vi "PV config A D input output.vi"(8 "error in (no error)":errorcluster, 9 "PV config A D input output - Cluster":T1={"Parameter"=enum." Configuration DO2 (019)", "Parameter\nread only<->describe"=FALSE, "off<->on   "=TRUE, "Configuration DO1 / DO2 / R1 / R2 / R3"=0, "Configuration AO1"=0, "Config. Acces. A1/A2"=0, "Config. Acces. B1/B2"=0, "Configuration DI1 / DI2 / DI3"=0} {"Configuration DI1 / DI2 / DI3" items=["0 = deactivated", "1 = enable venting", "2 = heating", "3 = sealing gas", "4 = run-up time control", "5 = rotation speed setting mode", "6 =", "7 = Sensor 1 HV enable"]; "Config. Acces. B1/B2" items=[" fan (continous operation) (default)", " venting valve, normally closed", " heating", " backing pump", " fan (temperature controlled)", " sealing gas", " always 0 (off)", " always 1 (on)", " power failure venting unit"]; "Config. Acces. A1/A2" items=[" fan (continous operation)", " venting valve, normally closed", " heating", " backing pump", " fan (temperature controlled)", " sealing gas", " always off", " always on", " power failure venting unit"]; "Configuration DO1 / DO2 / R1 / R2 / R3" items=["0 = rot. speed switch point attained", "1 = no error", "2 = error", "3 = warning", "4 = error and/or warning", "5 = set speed attained", "6 = pump on", "7 = pump accelerates", "8 = pump decelerater", "9 = always 0 (off)", "10 = always 1 (on)", "11 = remote priority active", "12 = heating", "13 = backing pump", "14 = sealing gas", "15 = pumping station", "16 = pump rotates", "17 = pump does not rotate", "18 = TMS temperature engaged  ", "19 = Pressure below pressure switchpoint 1", "20 = Pressure below pressure switchpoint 2"]; "Configuration AO1" items=["0 = actual rotation speed", "1 = power", "2 = current", "3 = always 0 V", "4 = always 10 V", "5 = follows AI1", "6 = Pressure value 1", "7 = Pressure value 2"]}, 10 "Adress of unit":u16=1 max=999 step=1, 11 "VISA session":refnum<visa-resource-name>) -> (0 "error out":errorcluster, 2 "response (data)":string, 3 "dup VISA session":refnum<visa-resource-name>)   [LabVIEW 2021, in "Pfeiffer Vacuum.lvlib"]
doc: "There are 15 parameters available, only one of which can be enabled at a time. \n\n Configuration DO2 (019)\n Configuration DO1 (024) \n Configuration heating output (032)\n Configuration accessory A1 (035)\n Configuration accessory B1 (036)\n Configuration accessory A2 (037)\n Configuration accessory B2 (038)\n Configuration Relais 1 (045)\n Configuration Relais 2 (046)\n Configuration Relais 3 (047)\n Configuration AO1 (055)\n Configuration AI1 (057)\n Configuration DI1 (062)\n Configuration DI2 (063)\n Configuration DI3 (064)\n\nNote: Any settings for an parameter that is not selected will be ignored. If a value is out of range, it will be changed to either the upper or the lower limit of the range."
uses:
  <instrlib>/Pfeiffer Vacuum/Pfeiffer Vacuum.lvlib
  <instrlib>/Pfeiffer Vacuum/Public/Turbopumps/PV config A D input output - Cluster.ctl
panel:
  # "<--------------                  ------------->     \n                                                                                        false                             true \n Configuration heating output K4    :                           heat/TMS            ealing gas valve control  \n Configuration AI 1                          :                            disabled                       set speed"
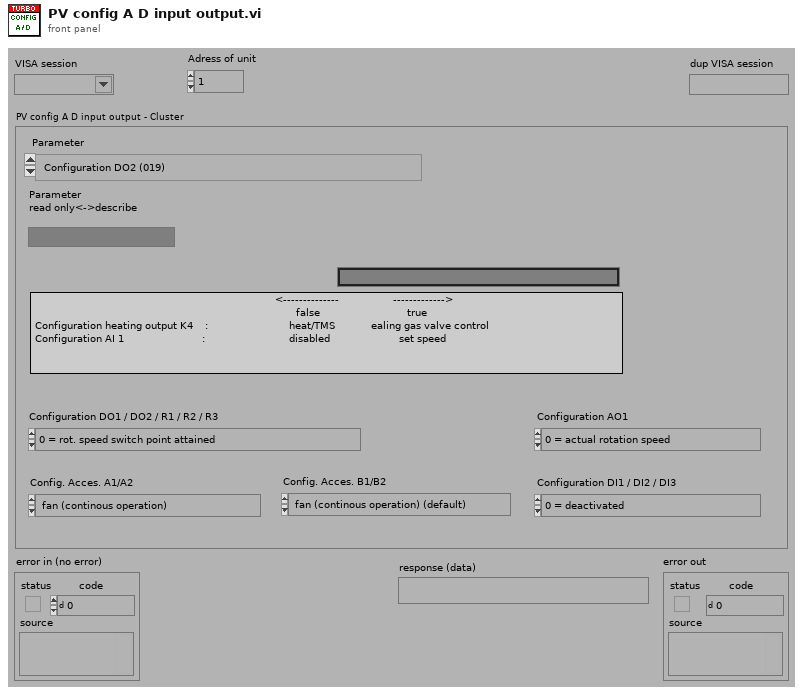
[diagram p1: front panel]
types:
  T1 = typedef "Pfeiffer Vacuum.lvlib/PV config A D input output - Cluster.ctl" = cluster{"Parameter":enum16{" Configuration DO2 (019)", " Configuration DO1 (024)", " Configuration heating output (032)", " Configuration accessory A1 (035)", " Configuration accessory B1 (036)", " Configuration accessory A2 (037)", " Configuration accessory B2 (038)", " Configuration Relais 1 (045)", " Configuration Relais 2 (046)", " Configuration Relais 3 (047)", " Configuration AO1 (055)", " Configuration AI1 (057)", " Configuration DI1 (062)", " Configuration DI2 (063)", " Configuration DI3 (064)"}, "Parameter\nread only<->describe":bool, "off<->on   ":bool, "Configuration DO1 / DO2 / R1 / R2 / R3":u16, "Configuration AO1":u16, "Config. Acces. A1/A2":u16, "Config. Acces. B1/B2":u16, "Configuration DI1 / DI2 / DI3":u16}
  T2 = enum16{" Configuration DO2 (019)", " Configuration DO1 (024)", " Configuration heating output (032)", " Configuration accessory A1 (035)", " Configuration accessory B1 (036)", " Configuration accessory A2 (037)", " Configuration accessory B2 (038)", " Configuration Relais 1 (045)", " Configuration Relais 2 (046)", " Configuration Relais 3 (047)", " Configuration AO1 (055)", " Configuration AI1 (057)", " Configuration DI1 (062)", " Configuration DI2 (063)", " Configuration DI3 (064)"}
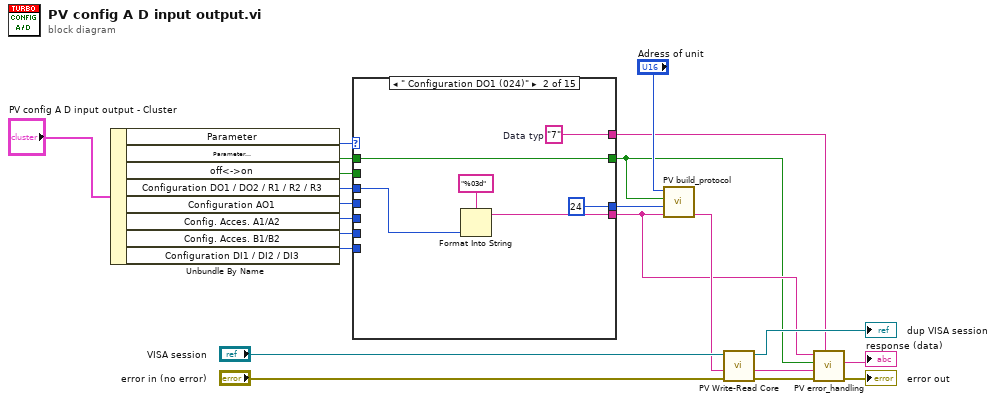
[diagram p0: block diagram]
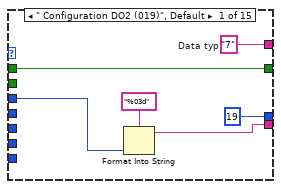
[diagram p2: hidden frame]
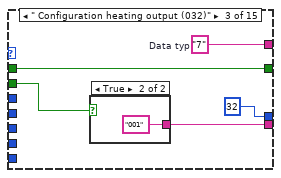
[diagram p3: hidden frame]
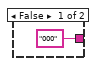
[diagram p4: hidden frame]
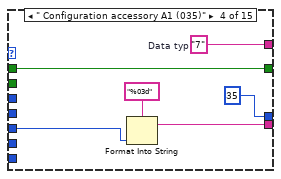
[diagram p5: hidden frame]
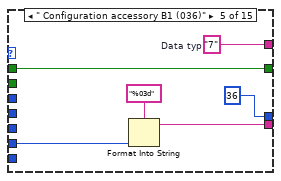
[diagram p6: hidden frame]
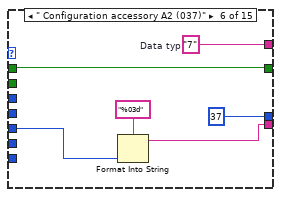
[diagram p7: hidden frame]
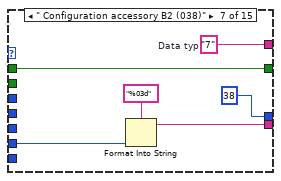
[diagram p8: hidden frame]
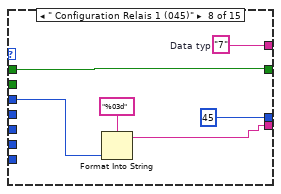
[diagram p9: hidden frame]
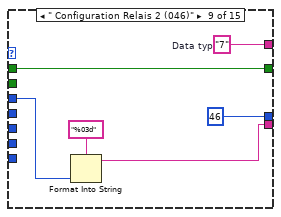
[diagram p10: hidden frame]
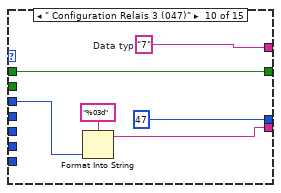
[diagram p11: hidden frame]
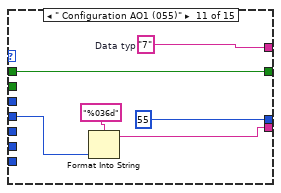
[diagram p12: hidden frame]
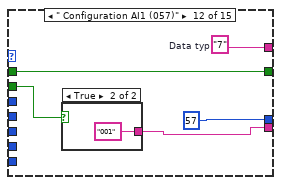
[diagram p13: hidden frame]
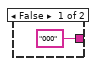
[diagram p14: hidden frame]
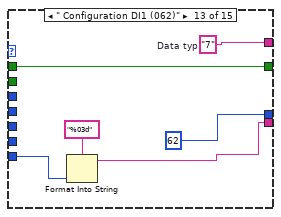
[diagram p15: hidden frame]
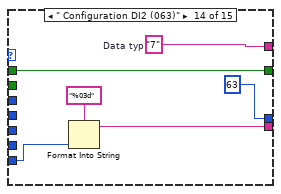
[diagram p16: hidden frame]
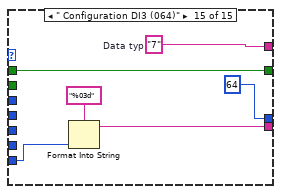
[diagram p17: hidden frame]
diagram:
  n1 = Unbundle By Name("PV config A D input output - Cluster") -> ("Parameter"=w9:T2, "Parameter\nread only<->describe"=w8:bool, "off<->on"=w7:bool, "Configuration DO1 / DO2 / R1 / R2 / R3"=w6:u16, "Configuration AO1"=w5:u16, "Config. Acces. A1/A2"=w4:u16, "Config. Acces. B1/B2"=w3:u16, "Configuration DI1 / DI2 / DI3"=w2:u16)
  n2 = case shown="\" Configuration DO1 (024)\"" w9 {
    tunnel: [u16 19 ("Parameter-number") u16 24 ("Parameter-number") u16 32 ("Parameter-number") u16 35 ("Parameter-number") u16 36 ("Parameter-number") u16 37 ("Parameter-number") u16 38 ("Parameter-number") u16 45 ("Parameter-number") u16 46 ("Parameter-number") u16 47 ("Parameter-number") u16 55 ("Parameter-number") u16 57 ("Parameter-number") u16 62 ("Parameter-number") u16 63 ("Parameter-number") u16 64 ("Parameter-number")] -> w21
    tunnel: [w24 w32 w38 w44 w52 w55 w60 w66 w73 w82 w88 w91 w98 w106 w112] -> w12
    tunnel: [w26 w30 w35 w42 w48 w57 w62 w69 w75 w78 w84 w93 w100 w103 w109] -> w11
    tunnel: [w27 w33 w37 w46 w50 w58 w63 w70 w76 w80 w86 w94 w101 w107 w113] -> w13
    tunnel: w8 -> [w26 w30 w35 w42 w48 w57 w62 w69 w75 w78 w84 w93 w100 w103 w109]
    tunnel: w7 -> [_ _ w36 _ _ _ _ _ _ _ _ w90 _ _ _]
    tunnel: w6 -> [w23 w29 _ _ _ _ _ w67 w72 w79 _ _ _ _ _]
    tunnel: w5 -> [_ _ _ _ _ _ _ _ _ _ w85 _ _ _ _]
    tunnel: w4 -> [_ _ _ w43 _ w54 _ _ _ _ _ _ _ _ _]
    tunnel: w3 -> [_ _ _ _ w49 _ w61 _ _ _ _ _ _ _ _]
    tunnel: w2 -> [_ _ _ _ _ _ _ _ _ _ _ _ w97 w104 w110]
    frame " Configuration DO2 (019)", Default {
      w27 = "7"  # Data typ
      n3 = Format Into String(format string="%03d" ("Format-String"), w23) -> (resulting string=w24:string)  [unwired: 2 in, 1 out]
    }
    frame " Configuration DO1 (024)" {
      w33 = "7"  # Data typ
      n4 = Format Into String(format string="%03d" ("Format-String"), w29) -> (resulting string=w32:string)  [unwired: 2 in, 1 out]
    }
    frame " Configuration heating output (032)" {
      w37 = "7"  # Data typ
      n5 = case shown="True" w36 {
        tunnel: ["000" ("Data") "001" ("Data")] -> w38
        frame False {
        }
        frame True {
        }
      }
    }
    frame " Configuration accessory A1 (035)" {
      w46 = "7"  # Data typ
      n6 = Format Into String(format string="%03d" ("Format-String"), w43) -> (resulting string=w44:string)  [unwired: 2 in, 1 out]
    }
    frame " Configuration accessory B1 (036)" {
      w50 = "7"  # Data typ
      n7 = Format Into String(format string="%03d" ("Format-String"), w49) -> (resulting string=w52:string)  [unwired: 2 in, 1 out]
    }
    frame " Configuration accessory A2 (037)" {
      w58 = "7"  # Data typ
      n8 = Format Into String(format string="%03d" ("Format-String"), w54) -> (resulting string=w55:string)  [unwired: 2 in, 1 out]
    }
    frame " Configuration accessory B2 (038)" {
      w63 = "7"  # Data typ
      n9 = Format Into String(format string="%03d" ("Format-String"), w61) -> (resulting string=w60:string)  [unwired: 2 in, 1 out]
    }
    frame " Configuration Relais 1 (045)" {
      w70 = "7"  # Data typ
      n10 = Format Into String(format string="%03d" ("Format-String"), w67) -> (resulting string=w66:string)  [unwired: 2 in, 1 out]
    }
    frame " Configuration Relais 2 (046)" {
      w76 = "7"  # Data typ
      n11 = Format Into String(format string="%03d" ("Format-String"), w72) -> (resulting string=w73:string)  [unwired: 2 in, 1 out]
    }
    frame " Configuration Relais 3 (047)" {
      w80 = "7"  # Data typ
      n12 = Format Into String(format string="%03d" ("Format-String"), w79) -> (resulting string=w82:string)  [unwired: 2 in, 1 out]
    }
    frame " Configuration AO1 (055)" {
      w86 = "7"  # Data typ
      n13 = Format Into String(format string="%036d" ("Format-String"), w85) -> (resulting string=w88:string)  [unwired: 2 in, 1 out]
    }
    frame " Configuration AI1 (057)" {
      w94 = "7"  # Data typ
      n14 = case shown="True" w90 {
        tunnel: ["000" ("Data") "001" ("Data")] -> w91
        frame False {
        }
        frame True {
        }
      }
    }
    frame " Configuration DI1 (062)" {
      w101 = "7"  # Data typ
      n15 = Format Into String(format string="%03d" ("Format-String"), w97) -> (resulting string=w98:string)  [unwired: 2 in, 1 out]
    }
    frame " Configuration DI2 (063)" {
      w107 = "7"  # Data typ
      n16 = Format Into String(format string="%03d" ("Format-String"), w104) -> (resulting string=w106:string)  [unwired: 2 in, 1 out]
    }
    frame " Configuration DI3 (064)" {
      w113 = "7"  # Data typ
      n17 = Format Into String(format string="%03d" ("Format-String"), w110) -> (resulting string=w112:string)  [unwired: 2 in, 1 out]
    }
  }
  n18 = call <instrlib>:"PV build_protocol.vi"("Data"=w12, "Parameter-number"=w21, "parameter\nread<->describe"=w11, "Adress"="Adress of unit") -> ("output"=w17:string)  [unwired: 3 in]
  n19 = call <instrlib>:"PV Write-Read Core.vi"("error in"="error in (no error)", "Write data in"=w17, "VISA session"="VISA session") -> ("error out"=w14:errorcluster, "response (data) out"=w15:string, "dup VISA session"=→"dup VISA session":refnum<visa-resource-name>)  [unwired: 2 in]
  n20 = call <instrlib>:"PV error_handling.vi"("Data Typ in"=w13, "error in"=w14, "response (data) in"=w15, "Parameter\nread only<->describe"=w11, "data in"=w12) -> ("error out"=→"error out":errorcluster, "Data out"=→"response (data)":string)  [unwired: 4 in, 1 out]
